vi "Add Default Child Node in Section.vi"(5 "Action":T2, 6 "Editable Nodes":T1(array[cluster]), 7 "Node Ref In":refnum<k20>, 9 "TypeName":string, 10 "Node Name":string, 11 "Parent Node":refnum<k20>) -> (1 "Cancelled?":bool, 2 "Updated Node Ref":refnum<k20>, 3 "Name out":string)   [LabVIEW 2025]
uses:
  Types/Section Child Node Types.ctl
  Types/Channel UI Controls.ctl
  Types/UserAction.ctl
panel:
  in  "Cancel":bool
  in  "Add/Save":bool
  in  "Name":string
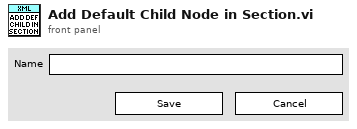
[diagram p1: front panel]
types:
  T1 = cluster{"Node":refnum<k20>, "Name":string, "Value":string}[]
  T2 = typedef "UserAction.ctl" = enum16{"Add", "Edit"}
  T3 = typedef "Section Child Node Types.ctl" = enum16{"Default Channel Node", "Default Section Node", "Default Waveform Node", "Dynamic Channel Node", "Dynamic Section Node", "Dynamic Waveform Node"}
  T4 = typedef "Channel UI Controls.ctl" = cluster{"Group Name":string, "Documentation":string, "Default Value":string, "Units":string, "Scalable":string, "Faultable":string, "Type Name":string, "Type ":string, "Name":string, "PropertyName":string}
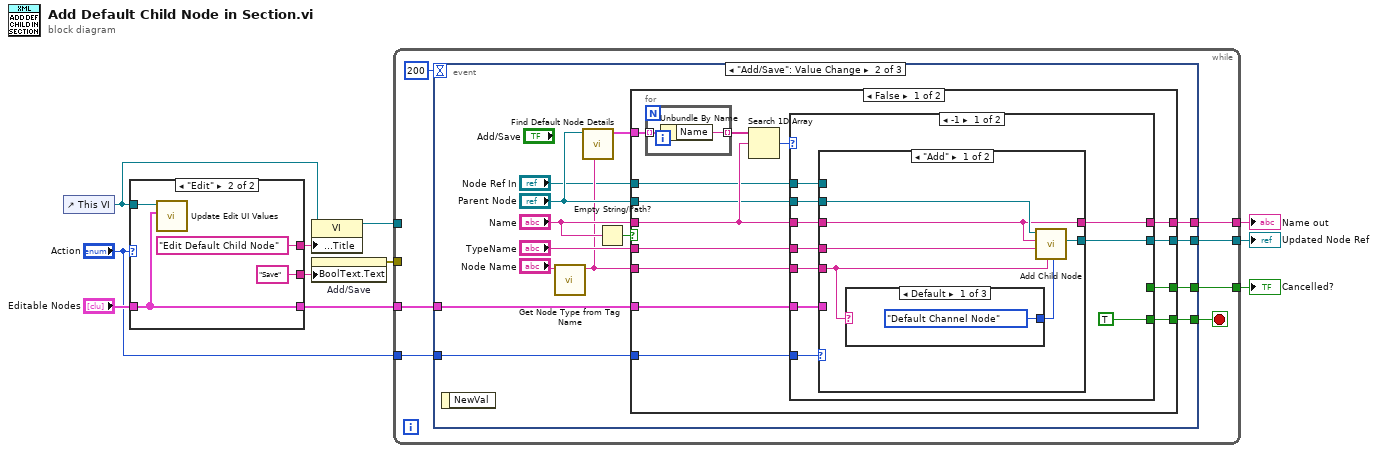
[diagram p0: block diagram]
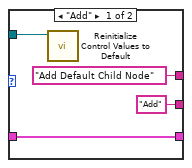
[diagram p2: hidden frame]
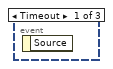
[diagram p3: hidden frame]
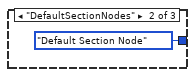
[diagram p4: hidden frame]
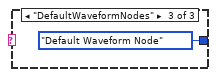
[diagram p5: hidden frame]
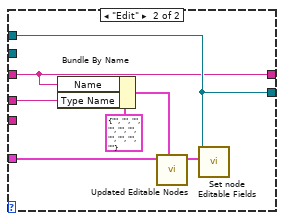
[diagram p6: hidden frame]
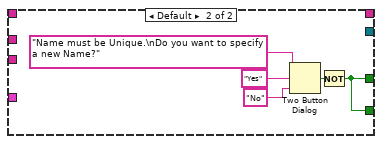
[diagram p7: hidden frame]
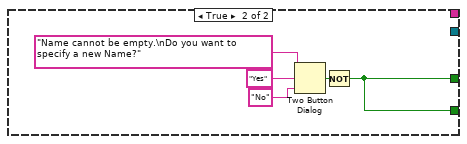
[diagram p8: hidden frame]
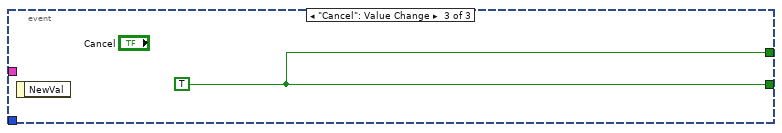
[diagram p9: hidden frame]
diagram:
  n1 = control-ref of="This VI"() -> (w6:refnum<vi>)
  n2 = case shown="\"Edit\"" "Action" {
    tunnel: "Editable Nodes" -> [w15 w18]
    tunnel: [w15 w18] -> w1
    tunnel: w6 -> [w14 w19]
    tunnel: ["Add" "Save"] -> w7
    tunnel: ["Add Default Child Node" "Edit Default Child Node"] -> w5
    frame "Add" {
      n3 = call "Reinitialize Control Values to Default.vi"("VI Ref"=w14) -> ()  [unwired: 10 in, 1 out]
    }
    frame "Edit" {
      n4 = call "Update Edit UI Values.vi"("Editable Nodes"=w18, "VI Ref"=w19) -> ()  [unwired: 9 in, 1 out]
    }
  }
  n5 = property class="VI"(reference=w6, "Front Panel.Title"=w5) -> (reference out=w3:refnum<vi>)  [unwired: 1 in, 1 out]
  n6 = property on="Add/Save" class="Bool"("BoolText.Text"=w7) -> (error out=w4:errorcluster)  [unwired: 2 in, 1 out]
  n7 = while {
    tunnel: [w26] -> w11
    tunnel: [w24] -> w10
    tunnel: [w22] -> w9
    tunnel: w4 -> [_]
    tunnel: w3 -> [_]
    tunnel: "Action" -> [w21]
    tunnel: w1 -> [w20]
    stop <- w23 stop-if-true
    n8 = event shown="[1] \"Add/Save\": Value Change" {
      selector: _ -> [_ _ _]
      dyn-events: _ -> [_ _ _]
      timeout: 200 -> [_ _ _]
      tunnel: [_ w39 _] -> w26
      tunnel: [_ w36 w93] -> w24
      tunnel: [_ w35 w93] -> w23
      tunnel: [_ w34 _] -> w22
      tunnel: w21 -> [_ w29 _]
      tunnel: w20 -> [_ w28 _]
      event Timeout {
        n9 = event-data() -> ()  [unwired: 1 in, 1 out]
      }
      event "Add/Save": Value Change {
        n10 = event-data() -> ()  [unwired: 1 in, 1 out]
        n11 = call "Get Node Type from Tag Name.vi"("Tag Name"="Node Name") -> ("Node Type"=w30:string)  [unwired: 9 in, 1 out]
        n12 = call "Find Default Node Details.vi"("Node Type"=w30, "Section Node"="Parent Node") -> ("Default Node Details"=w32:cluster{"Name":string, "TypeName":string}[])  [unwired: 8 in, 1 out]
        n13 = Empty String/Path?(string/path="Name") -> (empty?=w40:bool)
        n14 = case shown="False" w40 {
          tunnel: [w54 _] -> w39
          tunnel: "Name" -> [w53 _]
          tunnel: "TypeName" -> [w51 _]
          tunnel: [w50 w88] -> w36
          tunnel: [w49 w88] -> w35
          tunnel: [w48 _] -> w34
          tunnel: "Parent Node" -> [w47 _]
          tunnel: w32 -> [w46 _]
          tunnel: w30 -> [w44 _]
          tunnel: w29 -> [w43 _]
          tunnel: w28 -> [w42 _]
          tunnel: "Node Ref In" -> [w41 _]
          frame False {
            n15 = for {
              tunnel: w46 -> [w56] mode=indexing
              tunnel: [w55] -> w45 mode=indexing
              n16 = Unbundle By Name(w56) -> ("Name"=w55:string)
            }
            n17 = Search 1D Array(1D array=w45, element=w53) -> (index of element=w52:i32)  [unwired: 1 in]
            n18 = case shown="-1" w52 {
              tunnel: [w57 _] -> w54
              tunnel: w53 -> [w65 _]
              tunnel: w44 -> [w61 _]
              tunnel: w51 -> [w64 _]
              tunnel: [_ w83] -> w50
              tunnel: [TRUE w83] -> w49
              tunnel: [w63 _] -> w48
              tunnel: w47 -> [w62 _]
              tunnel: w43 -> [w60 _]
              tunnel: w42 -> [w59 _]
              tunnel: w41 -> [w58 _]
              frame -1 {
                n19 = case shown="\"Add\"" w60 {
                  tunnel: w65 -> [w67 w77]
                  tunnel: w64 -> [w72 w76]
                  tunnel: [w70 w78] -> w63
                  tunnel: w62 -> [w69 _]
                  tunnel: w61 -> [w68 _]
                  tunnel: w59 -> [_ w80]
                  tunnel: w58 -> [_ w78]
                  tunnel: [w67 w77] -> w57
                  frame "Add" {
                    n20 = case shown="Default" w68 {
                      tunnel: [Section_Child_Node_Types."Default Channel Node" ("Default Channel Type") Section_Child_Node_Types."Default Section Node" ("Default Channel Type") Section_Child_Node_Types."Default Waveform Node" ("Default Channel Type")] -> w71
                      frame Default {
                      }
                      frame "DefaultSectionNodes" {
                      }
                      frame "DefaultWaveformNodes" {
                      }
                    }
                    n21 = call "Add Child Node.vi"("Node Type"=w71, "Node Parent"=w68, "TypeName"=w72, "Name"=w67, "Parent Node"=w69) -> ("Updated Node Ref"=w70:refnum<k20>)  [unwired: 5 in, 1 out]
                  }
                  frame "Edit" {
                    n22 = Bundle By Name(cluster=T4 {"Group Name"="", "Documentation"="", "Default Value"="", "Units"="", "Scalable"="", "Faultable"="", "Type Name"="", "Type "="", "Name"="", "PropertyName"=""} ("Channel UI Controls"), "Name"=w77, "Type Name"=w76) -> (w81:T4)
                    n23 = call "Updated Editable Nodes.vi"("Channel UI Controls"=w81, "Editable Nodes"=w80) -> ("Updated Editable Nodes"=w79:T1)  [unwired: 9 in]
                    n24 = call "Set node Editable Fields.vi"("Editable Nodes"=w79, "Node In"=w78) -> ()  [unwired: 9 in, 1 out]
                  }
                }
              }
              frame Default {
                n25 = Two Button Dialog(message="Name must be Unique.\nDo you want to specify a new Name?" ("Errors"), 1:"No" ("F button name (\"Cancel\")"), 2:"Yes" ("T button name (\"OK\")")) -> (T button?=w84:bool)
                n26 = Not(x=w84) -> (.not. x?=w83:bool)
              }
            }
          }
          frame True {
            n27 = Two Button Dialog(message="Name cannot be empty.\nDo you want to specify a new Name?" ("Errors"), 1:"No" ("F button name (\"Cancel\")"), 2:"Yes" ("T button name (\"OK\")")) -> (T button?=w89:bool)
            n28 = Not(x=w89) -> (.not. x?=w88:bool)
          }
        }
      }
      event "Cancel": Value Change {
        w93 = TRUE
        n29 = event-data() -> ()  [unwired: 1 in, 1 out]
      }
    }
  }
  "Name out" <- w11
  "Cancelled?" <- w10
  "Updated Node Ref" <- w9
